vi "Get ListView Column Count.vi"(8 "error in (no error)":errorcluster caption="错误输入（无错误）", 11 "ListViewClass 输入":refnum<class "ListViewClass.lvclass"> caption="DNL_LabVIEW Object in") -> (0 "error out":errorcluster caption="错误输出", 2 "Count":i32, 3 "ListViewClass 输出":refnum<class "ListViewClass.lvclass"> caption="DNL_LabVIEW Object out")   [LabVIEW 2012, in "ListViewClass.lvclass"]
uses:
  ListViewClass.lvclass
  ListViewClass.lvclass/ListViewClass.ctl
  System.Windows.Forms
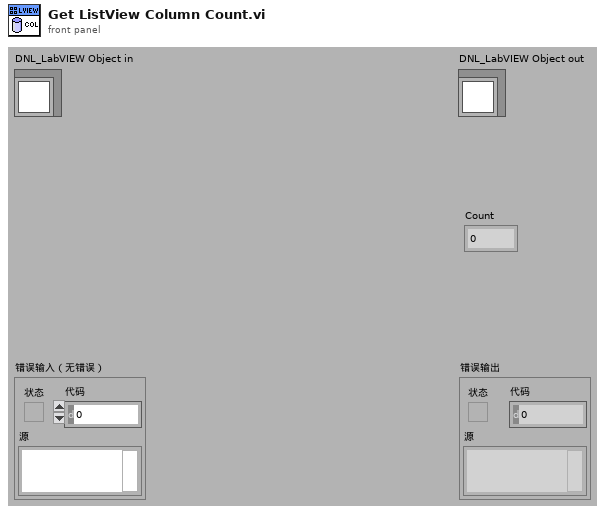
[diagram p1: front panel]
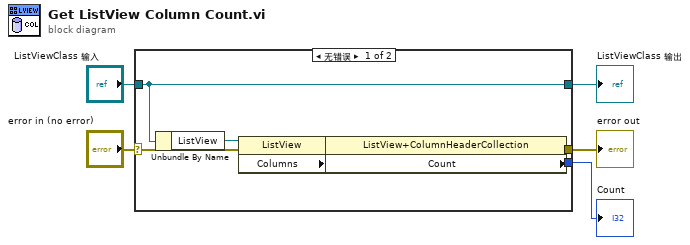
[diagram p0: block diagram]
diagram:
  n1 = case shown="无错误" "error in (no error)" {
    selector: "error in (no error)" -> [w9 w14]
    tunnel: [w6 w14] -> w4
    tunnel: [w12 w13] -> w2
    tunnel: "ListViewClass 输入" -> [w12 w13]
    tunnel: [w7 _] -> w1
    frame No Error {
      n2 = Unbundle By Name(w12) -> ("ListView"=w11:refnum<k24>)
      n3 = property class="ListView"(reference=w11, error in=w9) -> (error out=w8:errorcluster, "Columns"=w10:refnum<k24>)  [unwired: 1 out]
      n4 = property class="ListView+ColumnHeaderCollection"(reference=w10, error in=w8) -> (error out=w6:errorcluster, "Count"=w7:i32)  [unwired: 1 out]
    }
    frame Error {
    }
  }
  "error out" <- w4
  "ListViewClass 输出" <- w2
  "Count" <- w1
